vi "AP2_photoelectron_image_aquisition.vi"() -> ()   [LabVIEW 2023]
panel:
  in  "Tab Control 5":enum32{"Montoring"}(tab)
  out "A Counts":u32=157
  out "B Counts":u32
  out "A Counts/5F":dbl=3.0
  out "Avg Counts/F":dbl
  out "FPS":dbl=20.0 format="%#_2g"
  out "B Counts/5F":dbl
  out "Total Counts":u32=157
  out "T proc / ms":u32=50
  in  "Tab Control 4":enum32{"Raw Photoelectron Image"}(tab)
  out "Accumulated Image":i16[][](graph)
  in  "Tab Control 2":enum32{"Pixel Slice", "PES (MELEXIR)"}(tab)
  in  "Activate R Pix":bool
  in  "Center X":i32=500
  in  "Center Y":i32=500
  out "Pixel Slice":i32[](graph)
  in  "Activate PES":bool
  in  "Image Save Interval / s":dbl
  in  "Unit":u16(ring) items=["Pixel", "Electron Ek / eV", "Binding Energy / eV"]
  in  "Img Subtraction Mode":enum16{"A-B", "B-A", "A+B"}(ring)
  in  "PES Configuration file path":path
  in  "Detachment WL / nm":dbl
  out "PES Display":cluster{"Pixel":dbl[], "Intensity":dbl[]}(graph)
  in  "Tab Control":T1(tab)
  in  "Stop Control":bool
  in  "Save Image Button":bool
  in  "Discard Image Button":bool
  in  "Number of Images":u32=10000000
  in  "Frames/Update":i32=5
  in  "Frame timeout / ms":u32=1000
  in  "Buffers":u32=100
  in  "Region of interest":i32[](array[numeric])=[0, 0, 1020, 1020]
  in  "Threshold range":cluster{"Lower value":sgl, "Upper value":sgl}={"Lower value"=6.0, "Upper value"=1024.0}
  in  "Tuning Spline Path":path
  in  "Wavelength / nm":dbl
  out "Current Wavelength":dbl=0.77
  in  "Correction Factor / nm":dbl
  in  "Freq Doubled?":bool
  in  "Go to Wavelength":bool
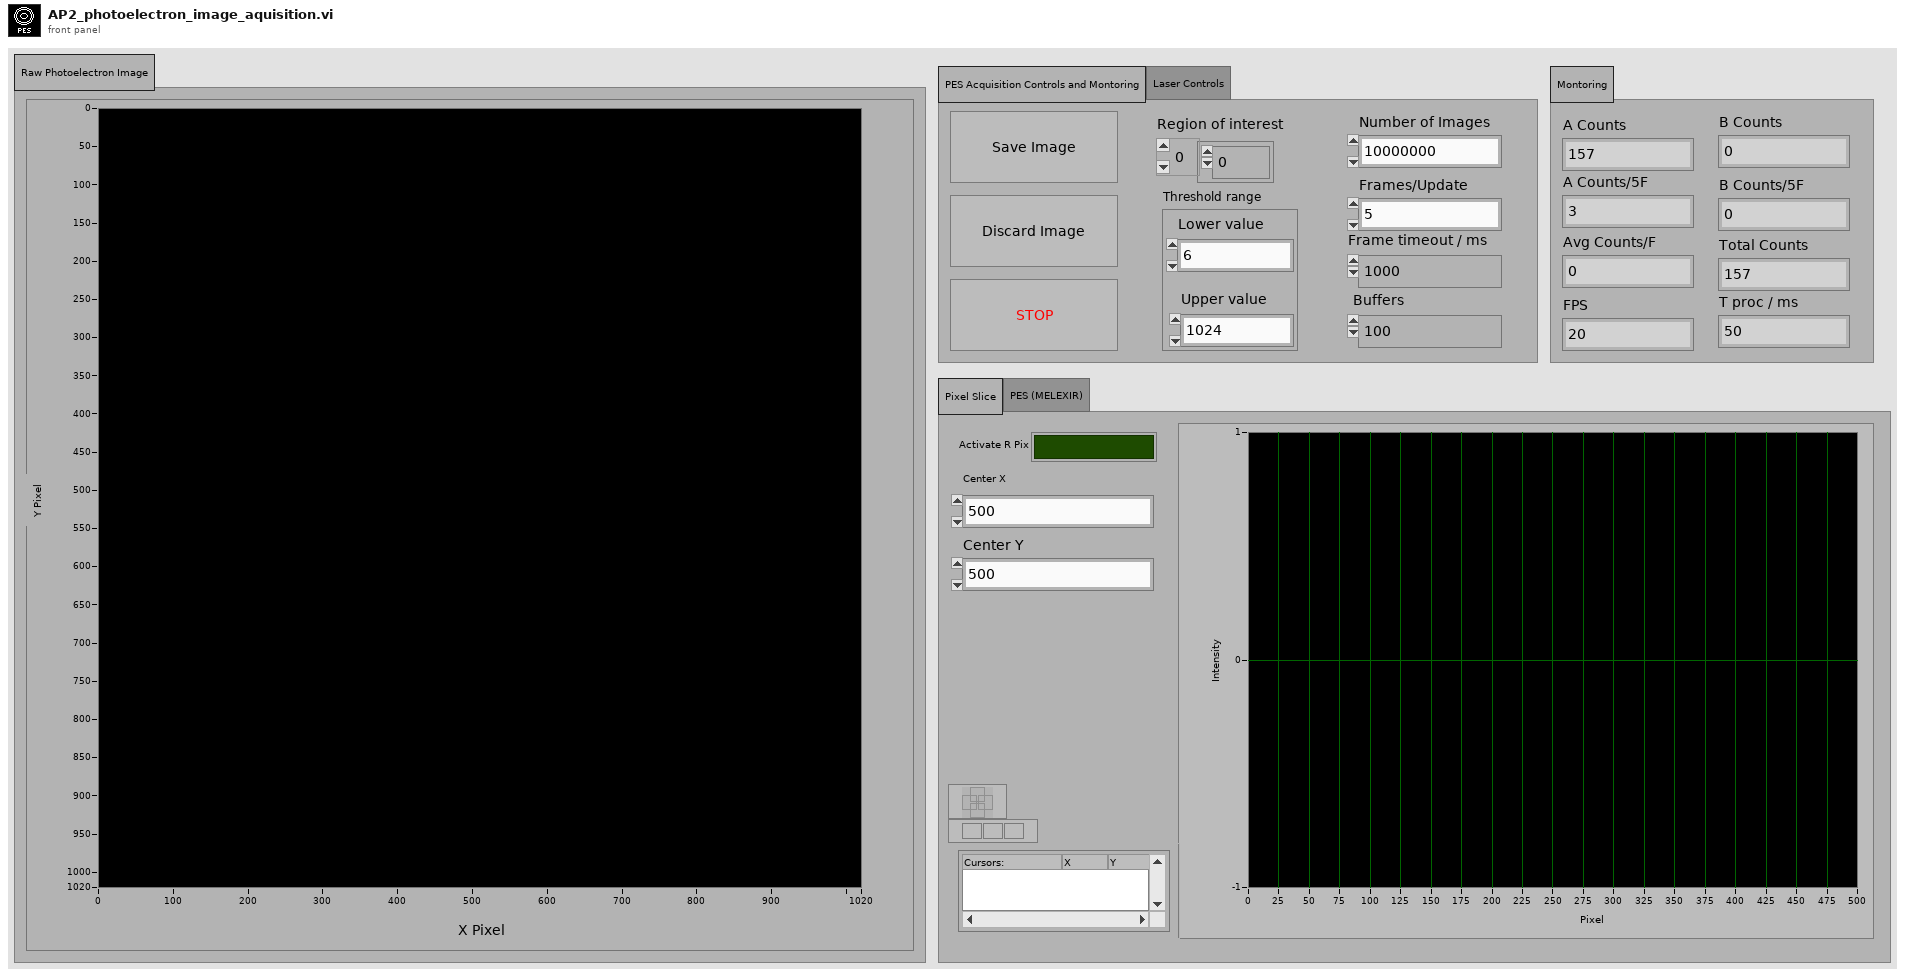
[diagram p1: front panel]
types:
  T1 = enum32{"PES Acquisition Controls and Montoring", "Laser Controls"}
  T2 = cluster{"Activate PES":bool, "Image Save Interval / s":dbl, "Unit":u16, "Img Subtraction Mode":enum16{"A-B", "B-A", "A+B"}, "Activate R Pix":bool, "Center x":i32, "Center y":i32, "Detachment Wavelength / nm":dbl, "Configuration file path":path}
  T3 = cluster{"A Counts":i32, "B Counts":i32, "Total Counts":i32, "A Counts / 5F":dbl, "B Counts / 5F":dbl, "Counts / F":dbl}
  T4 = cluster{"Region of interest":i32[], "Number of buffers":u32, "Frame timeout (ms)":u32}
  T5 = cluster{"queue out":refnum<queue>, "error out":errorcluster}
  T6 = cluster{"notifier out":refnum<notifier>, "error out":errorcluster}
  T7 = cluster{"A Counts":i32, "A Counts / 5F":dbl, "Update Counts?":bool, "Actual Width":u32, "B Counts / 5F ":dbl, "B Counts":i32, "Actual Height":u32, "Accumulated Image ":i16[][], "Total Counts":i32, "B Array i02":sgl[][], "A Array i01":sgl[][], "B Array":i16[][], "A Array":i16[][], "Region of interest":i32[], "Count Buffer Size 1":i32, "Init Img":i16[][], "counts /F":i16}
  T8 = cluster{"Frames/Update":i32, "Frames":i32, "Number of Images ":u32, "Threshold range":cluster{"Lower value":sgl, "Upper value":sgl}}
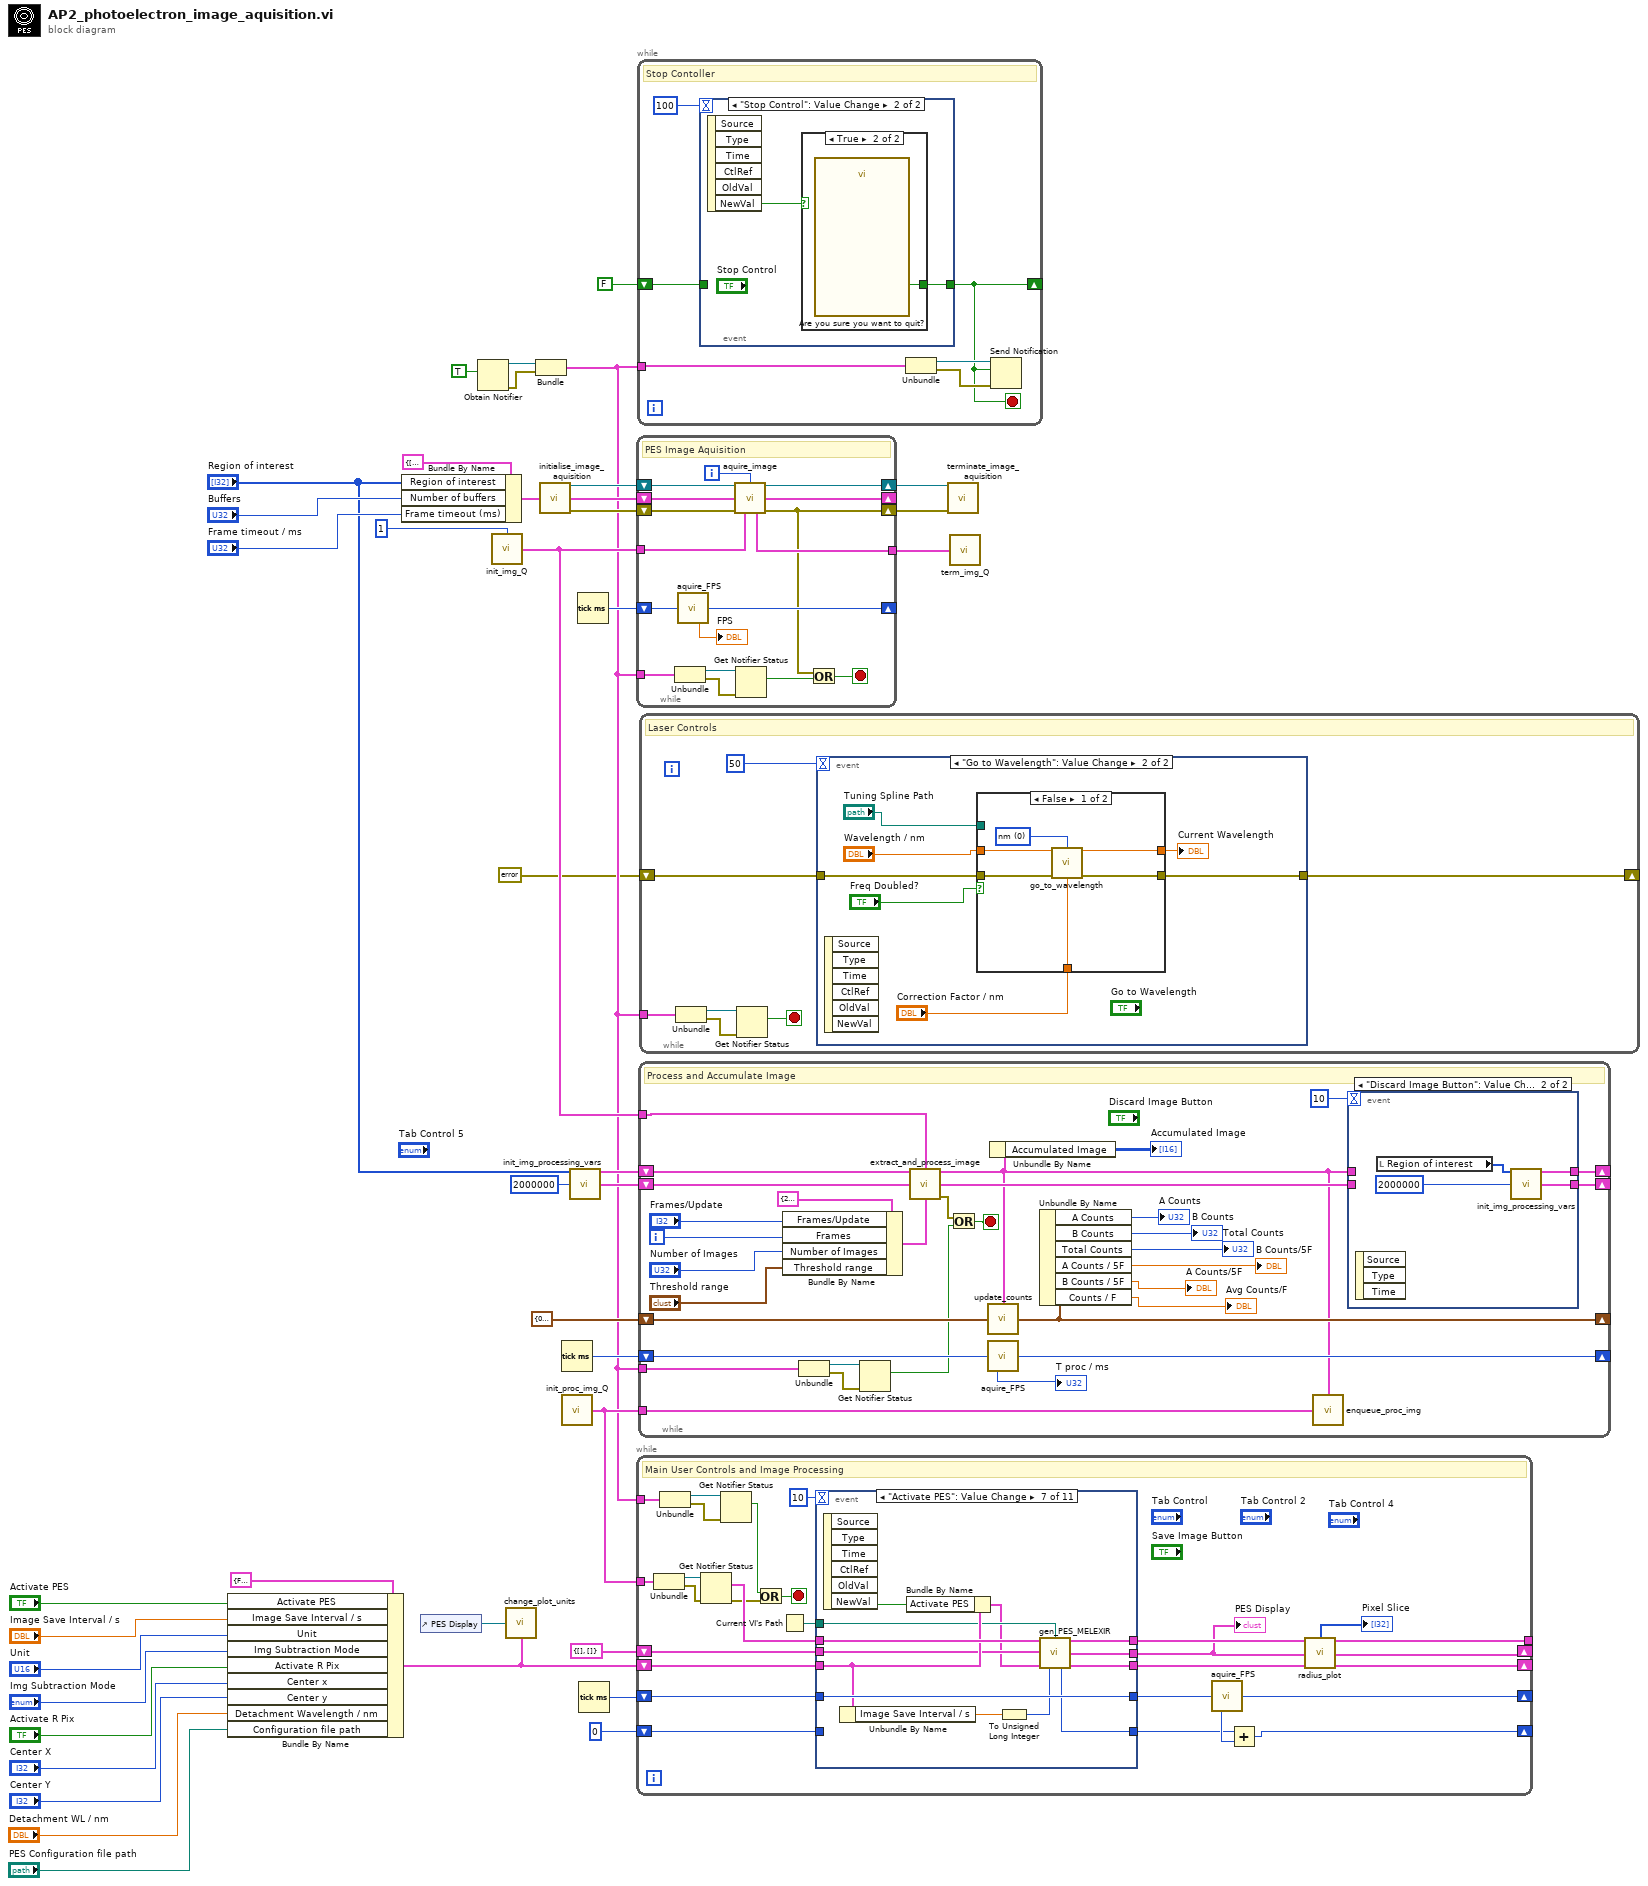
[diagram p0: block diagram]
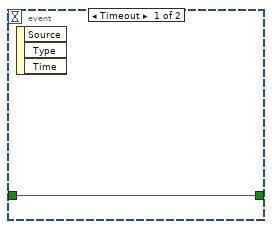
[diagram p2: hidden frame]
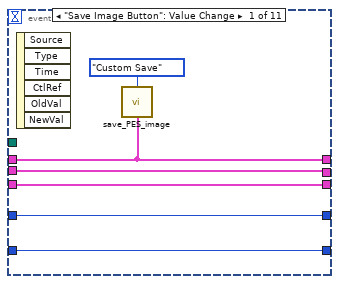
[diagram p4: hidden frame]
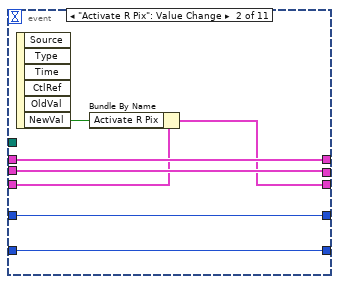
[diagram p5: hidden frame]
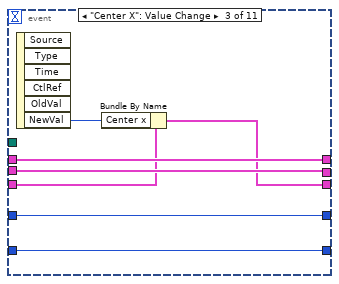
[diagram p6: hidden frame]
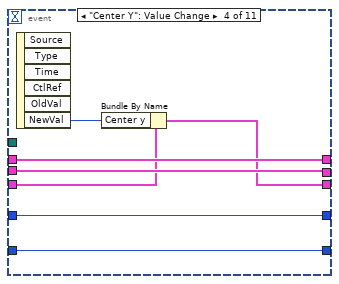
[diagram p7: hidden frame]
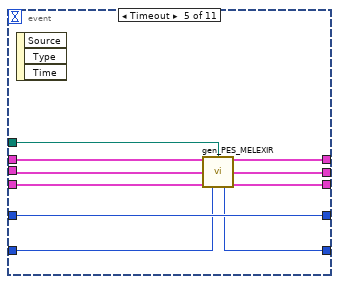
[diagram p8: hidden frame]
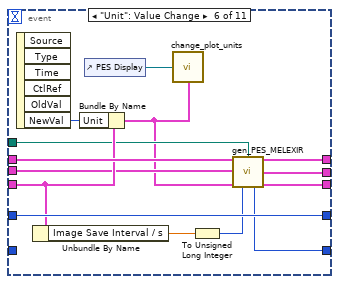
[diagram p9: hidden frame]
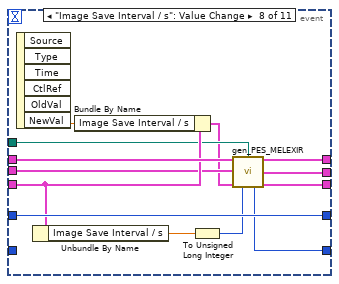
[diagram p10: hidden frame]
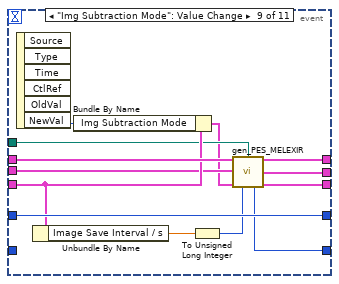
[diagram p11: hidden frame]
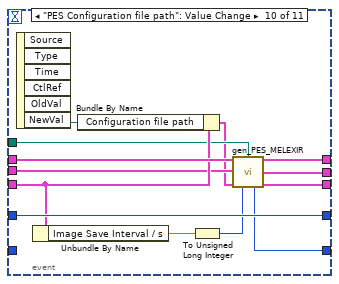
[diagram p12: hidden frame]
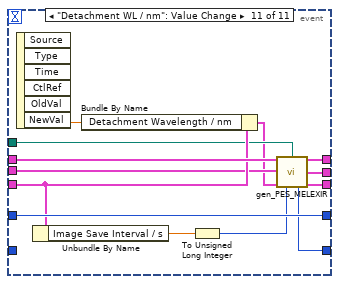
[diagram p13: hidden frame]
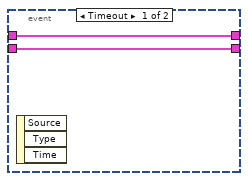
[diagram p14: hidden frame]
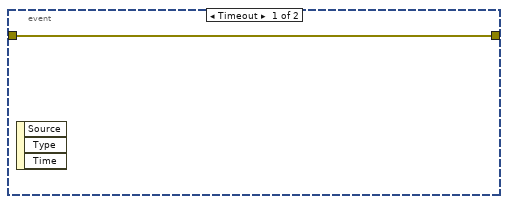
[diagram p15: hidden frame]
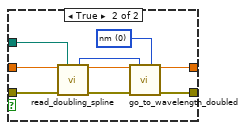
[diagram p16: hidden frame]
diagram:
  n1 = Bundle By Name(cluster=T2 {"Activate PES"=FALSE, "Image Save Interval / s"=2.0, "Unit"=2, "Img Subtraction Mode"=enum."A-B", "Activate R Pix"=FALSE, "Center x"=500, "Center y"=500, "Detachment Wavelength / nm"=0.0, "Configuration file path"=path ""}, "Activate PES"="Activate PES", "Image Save Interval / s"="Image Save Interval / s", "Unit"="Unit", "Img Subtraction Mode"="Img Subtraction Mode", "Activate R Pix"="Activate R Pix", "Center x"="Center X", "Center y"="Center Y", "Detachment Wavelength / nm"="Detachment WL / nm", "Configuration file path"="PES Configuration file path") -> (w7:T2)
  n2 = Bundle By Name(cluster=T4 {"Region of interest"=[], "Number of buffers"=0, "Frame timeout (ms)"=1000}, "Region of interest"="Region of interest", "Number of buffers"="Buffers", "Frame timeout (ms)"="Frame timeout / ms") -> (w36:T4)
  n3 = control-ref of="PES Display"() -> (w8:refnum<vi>)
  n4 = Obtain Notifier(notification data type=TRUE) -> (notifier out=w5:refnum<notifier>, error out=w4:errorcluster)  [unwired: 3 in, 1 out]
  n5 = call "init_img_Q.vi"("max queue size (-1, unlimited)"=1) -> ("Image Q Out"=w27:T5)  [unwired: 14 in]
  n6 = call "change_plot_units.vi"("PES Display Reference"=w8, "Controls"=w7) -> ()  [unwired: 14 in]
  n7 = Bundle("notifier out"=w5, "error out"=w4) -> (w3:T6)  [unwired: 1 in]
  n8 = call "initialise_image_aquisition.vi"("Imaging Variables In"=w36) -> ("IMAQ Session Out"=w41:refnum<k11>, "Imaging Variables Out"=w35:T4, "error out"=w40:errorcluster)  [unwired: 11 in, 1 out]
  n9 = Tick Count (ms)() -> (millisecond timer value=w15:u32)
  n10 = call "init_proc_img_Q.vi"() -> ("Proc Img Notifier Out"=w12:T6)  [unwired: 15 in]
  n11 = call "init_img_processing_vars.vi"("Region of interest"="Region of interest", "Count Buffer Size"=2000000 ("Count Buffer Size 1")) -> ("Image Data Out"=w24:T7, "Count Total Q Out"=w28:T5)  [unwired: 12 in]
  n12 = Tick Count (ms)() -> (millisecond timer value=w31:u32)
  n13 = Tick Count (ms)() -> (millisecond timer value=w14:u32)
  n14 = while {
    shift-right: [w58] -> w33
    shift-left: w41 -> [w56]
    shift-right: [w42] -> w32
    shift-left: w40 -> [w55]
    tunnel: w27 -> [w52]
    tunnel: [w51] -> w34
    shift-right: [w57] -> _
    shift-left: w35 -> [w53]
    shift-right: [w48] -> _
    shift-left: w31 -> [w50]
    tunnel: w3 -> [w45]
    i -> [w54]
    stop <- w43 stop-if-true
    # "PES Image Aquisition"
    n15 = Unbundle(w45) -> ("notifier out"=w46:refnum<notifier>, "error out"=w47:errorcluster)
    n16 = call "aquire_FPS.vi"("Time Value In /ms"=w50) -> ("Time Value Out /ms"=w48:u32, "FPS"=→"FPS":dbl)  [unwired: 12 in, 1 out]
    n17 = call "aquire_image.vi"("IMAQ Session In"=w56, "Buffer to extract"=w54, "Imaging Variables In"=w53, "error in (no error)"=w55, "Img Q Data In"=w52) -> ("IMAQ Session Out"=w58:refnum<k11>, "Imaging Variables Out"=w57:T4, "Img Q Data Out"=w51:T5, "error out"=w42:errorcluster)  [unwired: 7 in]
    n18 = Get Notifier Status(notifier=w46, error in (no error)=w47) -> (current notification=w44:bool)  [unwired: 4 out]
    n19 = Or(x=w42, y=w44) -> (x .or. y?=w43:bool)
  }
  n20 = while {
    tunnel: w3 -> [w83]
    tunnel: w12 -> [w74]
    shift-right: [w69] -> _
    shift-left: w7 -> [w81]
    shift-right: [w80] -> _
    shift-left: w14 -> [w79]
    shift-right: [w77] -> _
    shift-left: 0 -> [w78]
    shift-right: [w65] -> _
    shift-left: cluster{"Pixel":dbl[], "Intensity":dbl[]} {"Pixel"=[], "Intensity"=[]} ("PES Data") -> [w70]
    tunnel: [w68] -> _
    stop <- w61 stop-if-true
    # "Main User Controls and Image Processing"
    n21 = Unbundle(w74) -> ("notifier out"=w73:refnum<notifier>, "error out"=w72:errorcluster)
    n22 = Unbundle(w83) -> ("notifier out"=w85:refnum<notifier>, "error out"=w84:errorcluster)
    n23 = Get Notifier Status(notifier=w73, error in (no error)=w72) -> (current notification=w71:T7, error out=w59:errorcluster)  [unwired: 3 out]
    n24 = Get Notifier Status(notifier=w85, error in (no error)=w84) -> (current notification=w60:bool)  [unwired: 4 out]
    n25 = Or(x=w60, y=w59) -> (x .or. y?=w61:bool)
    n26 = Current VI's Path() -> (path=w62:path)
    n27 = event shown="[6] \"Activate PES\": Value Change" {
      selector: _ -> [_ _ _ _ _ _ _ _ _ _ _]
      dyn-events: _ -> [_ _ _ _ _ _ _ _ _ _ _]
      timeout: 10 -> [_ _ _ _ _ _ _ _ _ _ _]
      tunnel: w71 -> [w91 w98 w105 w112 w119 w134 w147 w160 w173 w186 w199]
      tunnel: [w91 w98 w105 w112 w121 w131 w144 w157 w170 w183 w196] -> w66
      tunnel: w81 -> [w89 w93 w100 w107 w118 w133 w146 w159 w172 w185 w198]
      tunnel: [w89 w92 w99 w106 w120 w130 w143 w156 w169 w182 w195] -> w63
      tunnel: w79 -> [w88 w97 w104 w111 w122 w136 w149 w162 w175 w188 w201]
      tunnel: [w88 w97 w104 w111 w122 w136 w149 w162 w175 w188 w201] -> w75
      tunnel: w78 -> [w87 w96 w103 w110 w115 _ _ _ _ _ _]
      tunnel: [w87 w96 w103 w110 w114 w127 w140 w153 w166 w179 w192] -> w64
      tunnel: [w86 w95 w102 w109 w116 w129 w142 w155 w168 w181 w194] -> w65
      tunnel: w70 -> [w86 w95 w102 w109 w117 w132 w145 w158 w171 w184 w197]
      tunnel: w62 -> [_ _ _ _ w113 w125 w138 w151 w164 w177 w190]
      event "Save Image Button": Value Change {
        n28 = event-data() -> ()  [unwired: 1 in, 6 out]
        n29 = call "save_PES_image.vi"("Save Type"=enum16{"Temp Img Save", "Custom Save"}."Custom Save", "Image Data In"=w91) -> ()  [unwired: 14 in]
      }
      event "Activate R Pix": Value Change {
        n30 = event-data() -> ("NewVal"=w94:bool)  [unwired: 1 in, 5 out]
        n31 = Bundle By Name(cluster=w93, "Activate R Pix"=w94) -> (w92:T2)
      }
      event "Center X": Value Change {
        n32 = event-data() -> ("NewVal"=w101:i32)  [unwired: 1 in, 5 out]
        n33 = Bundle By Name(cluster=w100, "Center x"=w101) -> (w99:T2)
      }
      event "Center Y": Value Change {
        n34 = event-data() -> ("NewVal"=w108:i32)  [unwired: 1 in, 5 out]
        n35 = Bundle By Name(cluster=w107, "Center y"=w108) -> (w106:T2)
      }
      event Timeout {
        n36 = event-data() -> ()  [unwired: 1 in, 3 out]
        n37 = call "gen_PES_MELEXIR.vi"("Img Data"=w119, "Current VI's Path"=w113, "PES Data In"=w117, "Controls"=w118, "Elapsed Time / ms"=w115) -> ("Img Data Out"=w121:T7, "PES Data"=w116:cluster{"Pixel":dbl[], "Intensity":dbl[]}, "Elapsed Time / ms Out"=w114:u32, "Controls Out"=w120:T2)  [unwired: 7 in]
      }
      event "Unit": Value Change {
        n38 = event-data() -> ("NewVal"=w135:u16)  [unwired: 1 in, 5 out]
        n39 = Unbundle By Name(w133) -> ("Image Save Interval / s"=w126:dbl)
        n40 = Bundle By Name(cluster=w133, "Unit"=w135) -> (w123:T2)
        n41 = control-ref of="PES Display"() -> (w124:refnum<vi>)
        n42 = call "change_plot_units.vi"("PES Display Reference"=w124, "Controls"=w123) -> ()  [unwired: 14 in]
        n43 = To Unsigned Long Integer(number=w126) -> (unsigned 32bit integer=w128:u32)
        n44 = call "gen_PES_MELEXIR.vi"("Img Data"=w134, "Current VI's Path"=w125, "PES Data In"=w132, "Controls"=w123, "Elapsed Time / ms"=w128) -> ("Img Data Out"=w131:T7, "PES Data"=w129:cluster{"Pixel":dbl[], "Intensity":dbl[]}, "Elapsed Time / ms Out"=w127:u32, "Controls Out"=w130:T2)  [unwired: 7 in]
      }
      event "Activate PES": Value Change {
        n45 = event-data() -> ("NewVal"=w148:bool)  [unwired: 1 in, 5 out]
        n46 = Unbundle By Name(w146) -> ("Image Save Interval / s"=w139:dbl)
        n47 = Bundle By Name(cluster=w146, "Activate PES"=w148) -> (w137:T2)
        n48 = To Unsigned Long Integer(number=w139) -> (unsigned 32bit integer=w141:u32)
        n49 = call "gen_PES_MELEXIR.vi"("Img Data"=w147, "Current VI's Path"=w138, "PES Data In"=w145, "Controls"=w137, "Elapsed Time / ms"=w141) -> ("Img Data Out"=w144:T7, "PES Data"=w142:cluster{"Pixel":dbl[], "Intensity":dbl[]}, "Elapsed Time / ms Out"=w140:u32, "Controls Out"=w143:T2)  [unwired: 7 in]
      }
      event "Image Save Interval / s": Value Change {
        n50 = event-data() -> ("NewVal"=w161:dbl)  [unwired: 1 in, 5 out]
        n51 = Unbundle By Name(w159) -> ("Image Save Interval / s"=w152:dbl)
        n52 = Bundle By Name(cluster=w159, "Image Save Interval / s"=w161) -> (w150:T2)
        n53 = To Unsigned Long Integer(number=w152) -> (unsigned 32bit integer=w154:u32)
        n54 = call "gen_PES_MELEXIR.vi"("Img Data"=w160, "Current VI's Path"=w151, "PES Data In"=w158, "Controls"=w150, "Elapsed Time / ms"=w154) -> ("Img Data Out"=w157:T7, "PES Data"=w155:cluster{"Pixel":dbl[], "Intensity":dbl[]}, "Elapsed Time / ms Out"=w153:u32, "Controls Out"=w156:T2)  [unwired: 7 in]
      }
      event "Img Subtraction Mode": Value Change {
        n55 = event-data() -> ("NewVal"=w174:enum16{"A-B", "B-A", "A+B"})  [unwired: 1 in, 5 out]
        n56 = Unbundle By Name(w172) -> ("Image Save Interval / s"=w165:dbl)
        n57 = Bundle By Name(cluster=w172, "Img Subtraction Mode"=w174) -> (w163:T2)
        n58 = To Unsigned Long Integer(number=w165) -> (unsigned 32bit integer=w167:u32)
        n59 = call "gen_PES_MELEXIR.vi"("Img Data"=w173, "Current VI's Path"=w164, "PES Data In"=w171, "Controls"=w163, "Elapsed Time / ms"=w167) -> ("Img Data Out"=w170:T7, "PES Data"=w168:cluster{"Pixel":dbl[], "Intensity":dbl[]}, "Elapsed Time / ms Out"=w166:u32, "Controls Out"=w169:T2)  [unwired: 7 in]
      }
      event "PES Configuration file path": Value Change {
        n60 = event-data() -> ("NewVal"=w187:path)  [unwired: 1 in, 5 out]
        n61 = Unbundle By Name(w185) -> ("Image Save Interval / s"=w178:dbl)
        n62 = Bundle By Name(cluster=w185, "Configuration file path"=w187) -> (w176:T2)
        n63 = To Unsigned Long Integer(number=w178) -> (unsigned 32bit integer=w180:u32)
        n64 = call "gen_PES_MELEXIR.vi"("Img Data"=w186, "Current VI's Path"=w177, "PES Data In"=w184, "Controls"=w176, "Elapsed Time / ms"=w180) -> ("Img Data Out"=w183:T7, "PES Data"=w181:cluster{"Pixel":dbl[], "Intensity":dbl[]}, "Elapsed Time / ms Out"=w179:u32, "Controls Out"=w182:T2)  [unwired: 7 in]
      }
      event "Detachment WL / nm": Value Change {
        n65 = event-data() -> ("NewVal"=w200:dbl)  [unwired: 1 in, 5 out]
        n66 = Unbundle By Name(w198) -> ("Image Save Interval / s"=w191:dbl)
        n67 = Bundle By Name(cluster=w198, "Detachment Wavelength / nm"=w200) -> (w189:T2)
        n68 = To Unsigned Long Integer(number=w191) -> (unsigned 32bit integer=w193:u32)
        n69 = call "gen_PES_MELEXIR.vi"("Img Data"=w199, "Current VI's Path"=w190, "PES Data In"=w197, "Controls"=w189, "Elapsed Time / ms"=w193) -> ("Img Data Out"=w196:T7, "PES Data"=w194:cluster{"Pixel":dbl[], "Intensity":dbl[]}, "Elapsed Time / ms Out"=w192:u32, "Controls Out"=w195:T2)  [unwired: 7 in]
      }
    }
    "PES Display" <- w65
    n70 = call "aquire_FPS.vi"("Time Value In /ms"=w75) -> ("Time Value Out /ms"=w80:u32, "Execution time / ms"=w76:u32)  [unwired: 12 in, 1 out]
    n71 = Add(x=w64, y=w76) -> (x+y=w77:u32)
    n72 = call "radius_plot.vi"("Img Data In"=w66, "Controls In"=w63) -> ("Integrated Intensity \n(Radias Direction)"=→"Pixel Slice":i32[], "Img Data Out"=w68:T7, "Controls Out"=w69:T2)  [unwired: 11 in]
  }
  n73 = while {
    tunnel: w3 -> [w205]
    shift-right: [w203] -> _
    shift-left: FALSE -> [w202]
    stop <- w203 stop-if-true
    # "Stop Contoller"
    n74 = event shown="[1] \"Stop Control\": Value Change" {
      selector: _ -> [_ _]
      dyn-events: _ -> [_ _]
      timeout: 100 -> [_ _]
      tunnel: [w208 w209] -> w203
      tunnel: w202 -> [w208 _]
      event Timeout {
        n75 = event-data() -> ()  [unwired: 1 in, 3 out]
      }
      event "Stop Control": Value Change {
        n76 = event-data() -> ("NewVal"=w210:bool)  [unwired: 1 in, 5 out]
        n77 = case shown="True" w210 {
          selector: w210 -> [w211 _]
          tunnel: [w211 w212] -> w209
          frame False {
          }
          frame True {
            n78 = call "Are you sure you want to quit?"() -> ("Yes"=w212:bool)  [unwired: 10 in, 1 out]
          }
        }
      }
    }
    n79 = Unbundle(w205) -> ("notifier out"=w206:refnum<notifier>, "error out"=w207:errorcluster)
    n80 = Send Notification(notification=w203, notifier=w206, error in (no error)=w207) -> ()  [unwired: 2 out]
  }
  n81 = while {
    shift-right: [w244] -> _
    shift-left: w15 -> [w245]
    shift-right: [w217] -> _
    shift-left: w24 -> [w216]
    shift-right: [w225] -> _
    shift-left: w28 -> [w242]
    tunnel: w27 -> [w240]
    shift-right: [w238] -> _
    shift-left: T3 {"A Counts"=0, "B Counts"=0, "Total Counts"=0, "A Counts / 5F"=0.0, "B Counts / 5F"=0.0, "Counts / F"=0.0} -> [w239]
    tunnel: w3 -> [w218]
    tunnel: w12 -> [w214]
    i -> [w228]
    stop <- w221 stop-if-true
    # "Process and Accumulate Image"
    n82 = Bundle By Name(cluster=T8 {"Frames/Update"=20, "Frames"=20, "Number of Images "=10000000, "Threshold range"={"Lower value"=6.0, "Upper value"=1024.0}}, "Frames/Update"="Frames/Update", "Frames"=w228, "Number of Images"="Number of Images", "Threshold range"="Threshold range") -> (w227:T8)
    n83 = Unbundle(w218) -> ("notifier out"=w223:refnum<notifier>, "error out"=w222:errorcluster)
    n84 = Get Notifier Status(notifier=w223, error in (no error)=w222) -> (current notification=w219:bool)  [unwired: 4 out]
    n85 = call "extract_and_process_image.vi"("Image Data In"=w216, "Raw Image Q In"=w240, "Count Total Q In"=w242, "Img Proc Controls in"=w227) -> ("Image Data Out"=w213:T7, "Count Total Q Out"=w226:T5, "error out"=w220:errorcluster)  [unwired: 9 in]
    n86 = Or(x=w220, y=w219) -> (x .or. y?=w221:bool)
    n87 = call "update_counts.vi"("Image Data In"=w213, "Count Display Data In"=w239) -> ("Count Display Data Out"=w238:T3)  [unwired: 13 in]
    n88 = call "aquire_FPS.vi"("Time Value In /ms"=w245) -> ("Time Value Out /ms"=w244:u32, "Execution time / ms"=→"T proc / ms":u32)  [unwired: 12 in, 1 out]
    n89 = Unbundle By Name(w213) -> ("Accumulated Image"=→"Accumulated Image":i16[][])
    n90 = Unbundle By Name(w238) -> ("A Counts"=→"A Counts":i32, "B Counts"=→"B Counts":i32, "Total Counts"=→"Total Counts":i32, "A Counts / 5F"=→"B Counts/5F":dbl, "B Counts / 5F"=→"A Counts/5F":dbl, "Counts / F"=→"Avg Counts/F":dbl)
    n91 = call "enqueue_proc_img.vi"("Proc Img Data In"=w213, "Proc Img Notifier In"=w214) -> ()  [unwired: 13 in, 1 out]
    n92 = event shown="[1] \"Discard Image Button\": Value Change" {
      selector: _ -> [_ _]
      dyn-events: _ -> [_ _]
      timeout: 10 -> [_ _]
      tunnel: w213 -> [w247 _]
      tunnel: [w247 w251] -> w217
      tunnel: w226 -> [w246 _]
      tunnel: [w246 w250] -> w225
      event Timeout {
        n93 = event-data() -> ()  [unwired: 1 in, 3 out]
      }
      event "Discard Image Button": Value Change {
        n94 = event-data() -> ()  [unwired: 1 in, 3 out]
        n95 = local read "Region of interest"() -> (w248:i32[])
        n96 = call "init_img_processing_vars.vi"("Region of interest"=w248, "Count Buffer Size"=2000000 ("Count Buffer Size 1")) -> ("Image Data Out"=w251:T7, "Count Total Q Out"=w250:T5)  [unwired: 12 in]
      }
    }
  }
  n97 = while {
    tunnel: w3 -> [w258]
    shift-right: [w252] -> _
    shift-left: errorcluster {"status"=FALSE, "code"=0, "source"=""} ("error out") -> [w253]
    stop <- w255 stop-if-true
    # "Laser Controls"
    n98 = Unbundle(w258) -> ("notifier out"=w257:refnum<notifier>, "error out"=w256:errorcluster)
    n99 = Get Notifier Status(notifier=w257, error in (no error)=w256) -> (current notification=w255:bool)  [unwired: 4 out]
    n100 = event shown="[1] \"Go to Wavelength\": Value Change" {
      selector: _ -> [_ _]
      dyn-events: _ -> [_ _]
      timeout: 50 -> [_ _]
      tunnel: w253 -> [w259 w266]
      tunnel: [w259 w265] -> w252
      event Timeout {
        n101 = event-data() -> ()  [unwired: 1 in, 3 out]
      }
      event "Go to Wavelength": Value Change {
        n102 = event-data() -> ()  [unwired: 1 in, 6 out]
        n103 = case shown="False" "Freq Doubled?" {
          tunnel: "Wavelength / nm" -> [w272 w279]
          tunnel: [w271 w281] -> w263
          tunnel: [w270 w280] -> w265
          tunnel: w266 -> [w269 w278]
          tunnel: "Tuning Spline Path" -> [_ w274]
          tunnel: "Correction Factor / nm" -> [w267 _]
          frame False {
            w268 = u16 0 items=["nm", "cm-1"] ("Unit")
            n104 = call "go_to_wavelength.vi"("Set Laser Position"=w272, "Unit"=w268, "error in (no error)"=w269, "Correction Factor /nm"=w267) -> ("Current Laser Position"=w271:dbl, "error out"=w270:errorcluster)  [unwired: 10 in]
          }
          frame True {
            w273 = u16 0 items=["nm", "cm-1"] ("Unit")
            n105 = call "read_doubling_spline.vi"("Wavelength"=w279, "Tuning Spline Path"=w274, "Error In"=w278) -> ("BBO Position"=w275:i32, "Wavelength Out"=w276:dbl, "Error Out"=w277:errorcluster)  [unwired: 10 in]
            n106 = call "go_to_wavelength_doubled.vi"("Set Laser Position"=w276, "Set BBO crystal position"=w275, "Unit"=w273, "error in (no error)"=w277) -> ("Current Laser Position"=w281:dbl, "error out"=w280:errorcluster)  [unwired: 10 in]
          }
        }
        "Current Wavelength" <- w263
      }
    }
  }
  n107 = call "terminate_image_aquisition.vi"("IMAQ Session In"=w33, "error in (no error)"=w32) -> ()  [unwired: 13 in, 1 out]
  n108 = call "term_img_Q.vi"("Image Q Out"=w34) -> ()  [unwired: 14 in, 1 out]
